vi "MultiD Array to 1D Array of VArrays.vi"(8 "error in (no error)":errorcluster, 10 "MultiD Array":variant) -> (0 "error out":errorcluster, 2 "Array of VArrays":variant[](array[variant]))   [LabVIEW 2020, in "JKI JSON Serialization.lvlib" / "JSON Serializer.lvclass"]
uses:
  JSON Serializer.lvclass
  <userlib>/_OpenG.lib/lvdata/lvdata.llb/openg_variant.lvlib
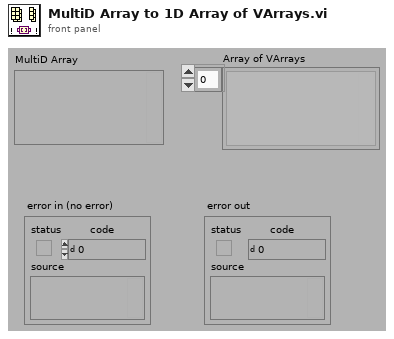
[diagram p1: front panel]
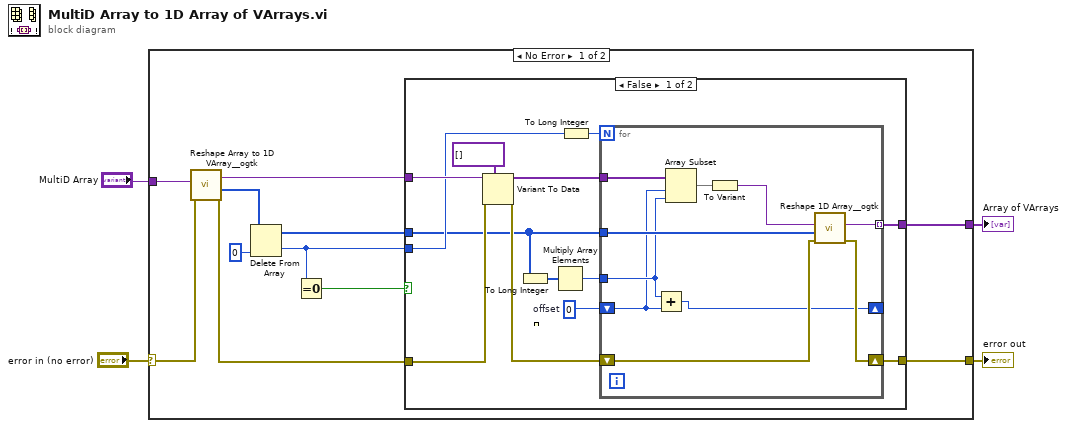
[diagram p0: block diagram]
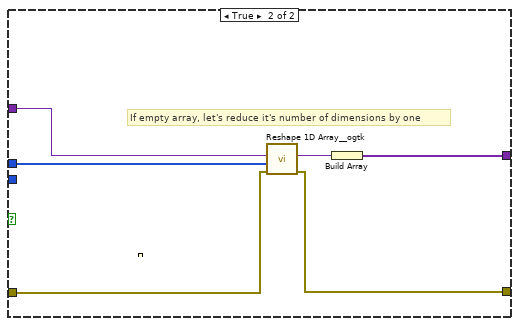
[diagram p2: hidden frame]
diagram:
  n1 = case shown="No Error" "error in (no error)" {
    selector: "error in (no error)" -> [w14 w45]
    tunnel: [w13 w45] -> w4
    tunnel: [w12 _] -> w1
    tunnel: "MultiD Array" -> [w15 _]
    frame No Error {
      n2 = call <userlib>:"Reshape Array to 1D VArray__ogtk.vi"("error in (no error)"=w14, "MultiD Array"=w15) -> ("error out"=w7:errorcluster, "Size(s)"=w9:u32[], "1D VArray"=w6:variant)  [unwired: 7 in]
      n3 = Delete From Array(array=w9, index=0) -> (deleted portion=w5:u32, array with subset deleted=w10:u32[])  [unwired: 1 in]
      n4 = Equal To 0?(x=w5) -> (x = 0?=w8:bool)
      n5 = case shown="False" w8 {
        tunnel: [w26 w44] -> w13
        tunnel: [w25 w42] -> w12
        tunnel: w10 -> [w18 w41]
        tunnel: w7 -> [w24 w39]
        tunnel: w6 -> [w23 w40]
        tunnel: w5 -> [w19 _]
        frame False {
          w28 = 0  # offset
          n6 = Variant To Data(error in=w24, type=variant[] [], Variant=w23) -> (data=w20:variant[], error out=w21:errorcluster)
          n7 = To Long Integer(number=w18) -> (32bit integer=w17:i32[])
          n8 = Multiply Array Elements(1:w17) -> (0:w27:i32)
          n9 = To Long Integer(number=w19) -> (32bit integer=w16:i32)
          n10 = for {
            N: w16 -> [_]
            tunnel: w18 -> [w38]
            tunnel: w20 -> [w34]
            shift-right: [w36] -> w26
            shift-left: w21 -> [w37]
            shift-right: [w35] -> _
            shift-left: w28 -> [w31]
            tunnel: w27 -> [w32]
            tunnel: [w30] -> w25 mode=indexing
            n11 = Add(x=w32, y=w31) -> (x+y=w35:i32)
            n12 = Array Subset(array=w34, index=w31, length=w32) -> (w33:variant[])
            n13 = To Variant(anything=w33) -> (Variant=w29:variant)
            n14 = call <userlib>:"Reshape 1D Array__ogtk.vi"("error in (no error)"=w37, "Size(s)"=w38, "1D Array"=w29) -> ("error out"=w36:errorcluster, "Reshaped VArray"=w30:variant)  [unwired: 7 in]
          }
        }
        frame True {
          # "If empty array, let's reduce it's number of dimensions by one"
          n15 = call <userlib>:"Reshape 1D Array__ogtk.vi"("error in (no error)"=w39, "Size(s)"=w41, "1D Array"=w40) -> ("error out"=w44:errorcluster, "Reshaped VArray"=w43:variant)  [unwired: 7 in]
          n16 = Build Array(w43) -> (w42:variant[])
        }
      }
    }
    frame Error {
    }
  }
  "error out" <- w4
  "Array of VArrays" <- w1
